vi "Application Name--constant.vi"() -> (3 "Application Name":string)   [LabVIEW 2020, in "Application.lvlib"]
doc: "Return the Application name.\n_____\nBased on DQMH Project Template 6.1.0.93."
uses:
  Application.lvlib
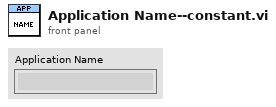
[diagram p1: front panel]
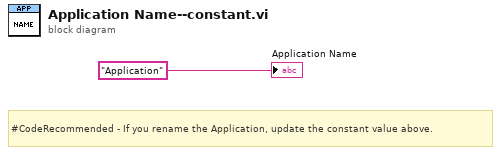
[diagram p0: block diagram]
diagram:
  # "#CodeRecommended - If you rename the Application, update the constant value above."
  "Application Name" <- "Application" ("Application Name 2")
